vi "Controller Convert PID Parameters to Coefficients.vi"(9 "Period":dbl, 10 "Derivative Time":dbl, 11 "Integral Time":dbl) -> (2 "Scaling Gain":dbl, 3 "PS Filter Coefficients":dbl[](array[numeric]))   [LabVIEW 2011, in "Controller VIs.lvlib"]
uses:
  Controller VIs.lvlib
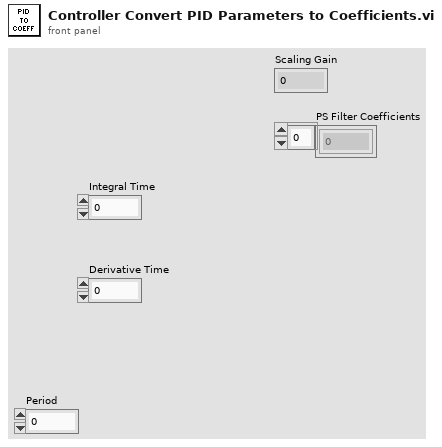
[diagram p1: front panel]
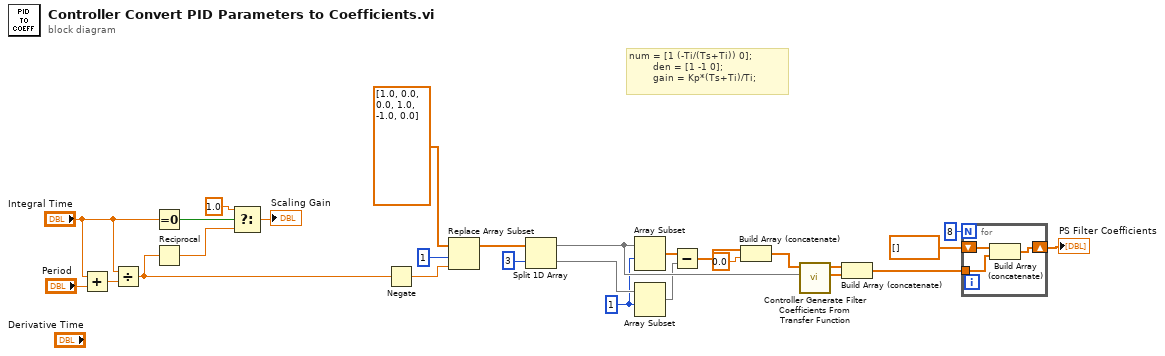
[diagram p0: block diagram]
diagram:
  w3 = 1 ("index")
  # "num = [1 (-Ti/(Ts+Ti)) 0];\n        den = [1 -1 0];\n        gain = Kp*(Ts+Ti)/Ti;"
  n1 = Add(x="Integral Time", y="Period") -> (x+y=w14:dbl)
  n2 = Divide(x="Integral Time", y=w14) -> (x/y=w15:dbl)
  n3 = Equal To 0?(x="Integral Time") -> (x = 0?=w20:bool)
  n4 = Reciprocal(x=w15) -> (1/x=w17:dbl)
  n5 = Select(t=1.0, s=w20, f=w17) -> (s? t:f=→"Scaling Gain":dbl)
  n6 = Negate(x=w15) -> (-x=w16:dbl)
  n7 = Replace Array Subset(array=dbl[] [1.0, 0.0, 0.0, 1.0, -1.0, 0.0] ("coeffs"), new element=w16, index=1) -> (w22:dbl[])
  n8 = Split 1D Array(array=w22, index=3) -> (first subarray=w27:dbl[], second subarray=w25:dbl[])
  n9 = Array Subset(array=w27, index=w3) -> (w5:dbl[])  [unwired: 1 in]
  n10 = Array Subset(array=w25, index=w3) -> (w4:dbl[])  [unwired: 1 in]
  n11 = Subtract(x=w5, y=w4) -> (x-y=w7:dbl[])
  n12 = Build Array (concatenate)(w7, 0.0 ("Numeric")) -> (w26:dbl[])
  n13 = call "Controller Generate Filter Coefficients From Transfer Function.vi"("denominator"=w27, "numerator"=w26) -> ("coeff a"=w1:dbl[], "coeff b"=w2:dbl[])  [unwired: 7 in, 1 out]
  n14 = Build Array (concatenate)(w2, w1) -> (w23:dbl[])
  n15 = for {
    N: 8 -> [_]
    tunnel: w23 -> [w29]
    shift-right: [w28] -> w12
    shift-left: dbl[] [] ("Array") -> [w30]
    n16 = Build Array (concatenate)(w30, w29) -> (w28:dbl[])
  }
  "PS Filter Coefficients" <- w12
